vi "Get Item Icon.vi"(8 "error in (no error)":errorcluster, 11 "VI in":refnum<class "VI.lvclass">) -> (0 "error out":errorcluster, 3 "VI out":refnum<class "VI.lvclass">)   [LabVIEW 2020, in "VI Properties Editor.lvlib" / "VI.lvclass"]
doc: "Gets the icon for <B>VI in</B>."
uses:
  VI.lvclass
  VI.lvclass/VI.ctl
  <vilib>/LabVIEW Icon API/lv_icon/Controls/Alignment.ctl
  <vilib>/LabVIEW Icon API/lv_icon/Controls/Font.ctl
  <vilib>/LabVIEW Icon API/lv_icon/Controls/BodyText.ctl
  <vilib>/LabVIEW Icon API/lv_icon/lv_icon.lvlib
  <vilib>/LabVIEW Icon API/LabVIEW Icon API.lvlib
  VI Properties Editor.lvlib
panel:
  in  "Localized string template":string="Template"
  in  "Localied string text":string="Text"
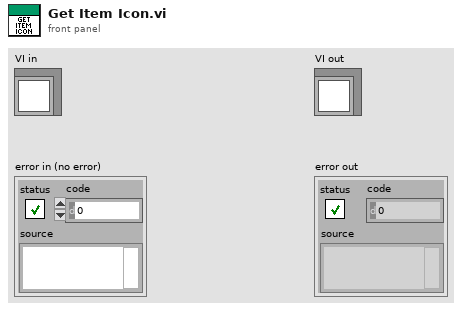
[diagram p1: front panel]
types:
  T1 = typedef "BodyText.ctl" = cluster{"Line 1 text":string, "Line 2 text":string, "Line 3 text":string, "Line 4 text":string, "Line 1 color":u32, "Line 2 color":u32, "Line 3 color":u32, "Line 4 color":u32, "Body Text Spec":cluster{"Font":T2, "Alignment":T3, "Size":u8}, "Center text vertically":bool, "Capitalize Text":bool}
  T2 = typedef "Font.ctl" = string
  T3 = typedef "Alignment.ctl" = u16
  T4 = typedef "LabVIEW Icon Stored Information.ctl" = cluster{"Text Visible?":bool, "Text Opacity":u8, "Templ Visible?":bool, "Templ Opacity":u8, "Relative Path from 1 to 2":path, "Image":picture, "All User Layers":refnum<class "Layer.lvclass">[], "Body Text":T1}
  T5 = typedef "imagedata.ctl" = cluster{"image type":i32, "image depth":i32, "image":u8[], "mask":u8[], "colors":u32[], "Rectangle":cluster{"left":i16, "top":i16, "right":i16, "bottom":i16}}
  T6 = typedef "Layer.ctl" = cluster{"LayerIcon":picture, "LayerName":string, "Opacity":u8, "Visibility?":bool}
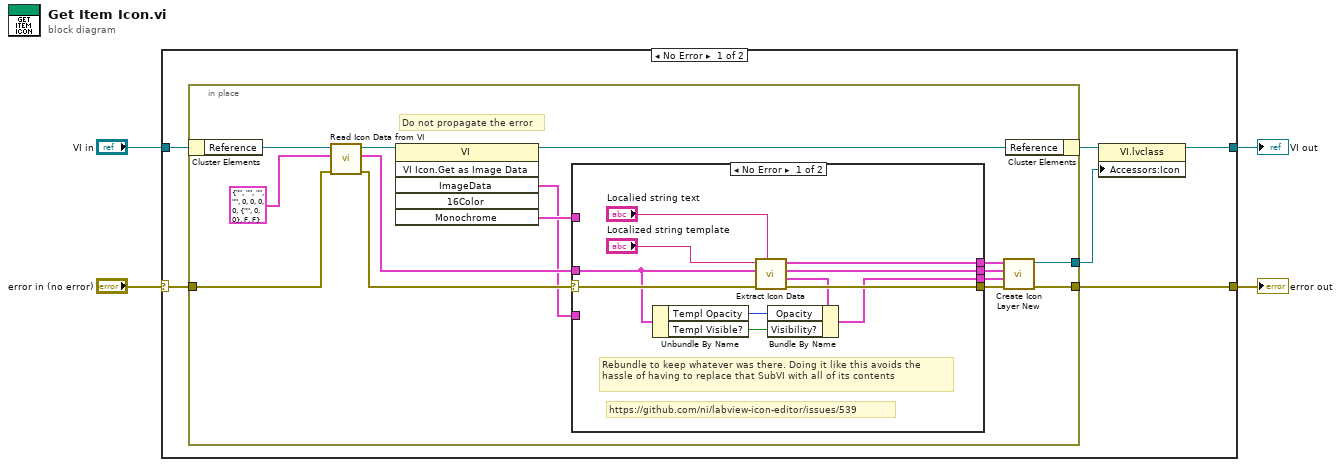
[diagram p0: block diagram]
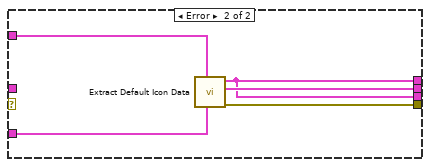
[diagram p2: hidden frame]
diagram:
  n1 = case shown="No Error" "error in (no error)" {
    selector: "error in (no error)" -> [w9 w41]
    tunnel: "VI in" -> [w10 w42]
    tunnel: [w8 w41] -> w2
    tunnel: [w5 w42] -> w1
    frame No Error {
      n2 = in-place {
        in-place-border: w9 -> [w23]
        in-place-border: [w12] -> w8
        in-place-border: [w11] -> w6
        # "Do not propagate the error"
        n3 = in-place-cluster #1(w10) -> ("Reference"=w25:refnum<vi>)
        n4 = call <vilib>:"Read Icon Data from VI.vi"("error in (no error)"=w23, "Default body text"=T1 {"Line 1 text"="", "Line 2 text"="", "Line 3 text"="", "Line 4 text"="", "Line 1 color"=0, "Line 2 color"=0, "Line 3 color"=0, "Line 4 color"=0, "Body Text Spec"={"Font"="", "Alignment"=0, "Size"=0}, "Center text vertically"=FALSE, "Capitalize Text"=FALSE}, "VI Ref in"=w25) -> ("error out"=w20:errorcluster, "Data"=w19:T4, "VI Ref out"=w21:refnum<vi>)  [unwired: 6 in]
        n5 = invoke class="VI" method="VI Icon.Get as Image Data"(reference=w21) -> (reference out=w24:refnum<vi>, "ImageData"=w17:T5, "Monochrome"=w18:T5)  [unwired: 5 in, 3 out]
        n6 = case shown="No Error" w20 {
          selector: w20 -> [w35 _]
          tunnel: [w35 w39] -> w16
          tunnel: w19 -> [w29 _]
          tunnel: [w33 w37] -> w13
          tunnel: [w32 w40] -> w14
          tunnel: [w26 w37] -> w15
          tunnel: w17 -> [_ w38]
          tunnel: w18 -> [_ w36]
          frame No Error {
            # "https://github.com/ni/labview-icon-editor/issues/539"
            # "Rebundle to keep whatever was there. Doing it like this avoids the hassle of having to replace that SubVI with all of its contents"
            n7 = Unbundle By Name(w29) -> ("Templ Opacity"=w28:u8, "Templ Visible?"=w27:bool)
            n8 = call <vilib>:"Extract Icon Data.vi"("Text layer name"="Localied string text", "Icon data in"=w29, "Template layer name"="Localized string template") -> ("Template data"=w30:T6, "Icon data out"=w32:T4, "Text data"=w33:T6)  [unwired: 5 in, 1 out]
            n9 = Bundle By Name(cluster=w30, "Opacity"=w28, "Visibility?"=w27) -> (w26:T6)
          }
          frame Error {
            n10 = call <vilib>:"Extract Default Icon Data.vi"("Color Icon"=w38, "BW Icon"=w36) -> ("error out"=w39:errorcluster, "VI Icon Data out"=w40:T4, "Default Icon Template data"=w37:T6)  [unwired: 7 in]
          }
        }
        n11 = call "Create Icon Layer New.vi"("error in (no error)"=w16, "Template data"=w15, "Icon data"=w14, "Text data"=w13) -> ("error out"=w12:errorcluster, "Icon out"=w11:refnum<class "Icon.lvclass">)  [unwired: 6 in]
        n12 = in-place-cluster #1("Reference"=w24) -> (w7:refnum<class "VI.lvclass">)
      }
      n13 = property class="VI.lvclass"(reference=w7, "Accessors:Icon"=w6) -> (reference out=w5:refnum<class "VI.lvclass">)  [unwired: 1 in, 1 out]
    }
    frame Error {
    }
  }
  "error out" <- w2
  "VI out" <- w1
